vi "Get Heater.vi"(8 "error in (no error)":errorcluster, 9 "Heater Start Btn":refnum<vi>, 10 "Digital in":refnum<vi>, 11 "data":T1 {"Rotate_IND" items=["стоп", "Качалка Режим Авто", "Качалка Режим Ручной"]; "Termex_IND" items=["Термостат старт"=1, "Термостат стоп"=0]; "Mix_IND" items=["Мешалка движение вперёд"=1, "Мешалка движение назад"=2, "Мешалка стоп"=0]}) -> (0 "error out":errorcluster)   [LabVIEW 2023, in "GUI.lvlib" / "gui.lvclass"]
uses:
  gui.lvclass
  gui.lvclass/gui.ctl
  Modbus PLC/Modbus PLC/Data.ctl
  Modbus PLC/Modbus PLC/Modbus PLC.lvclass
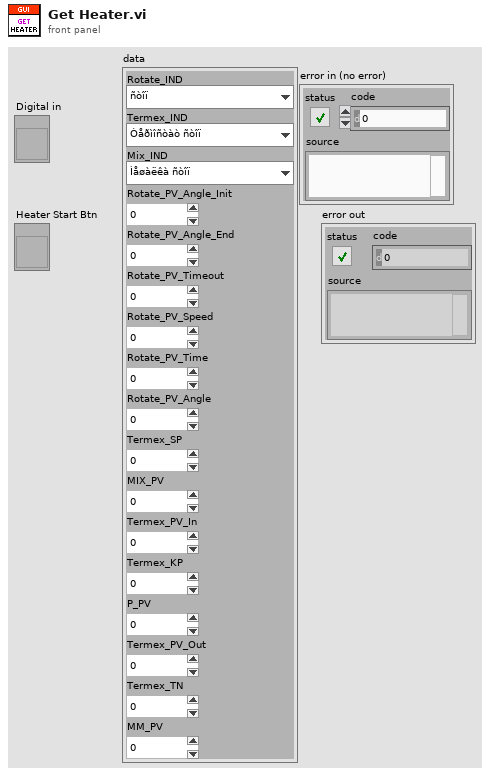
[diagram p1: front panel]
types:
  T1 = typedef "Modbus PLC.lvlib/Modbus PLC.lvclass/Data.ctl" = cluster{"Rotate_IND":u16, "Termex_IND":u16, "Mix_IND":u16, "Rotate_PV_Angle_Init":u16, "Rotate_PV_Angle_End":u16, "Rotate_PV_Timeout":u16, "Rotate_PV_Speed":u16, "Rotate_PV_Time":u16, "Rotate_PV_Angle":u16, "Termex_SP":sgl, "MIX_PV":u16, "Termex_PV_In":sgl, "Termex_KP":sgl, "P_PV":sgl, "Termex_PV_Out":sgl, "Termex_TN":sgl, "MM_PV":sgl}
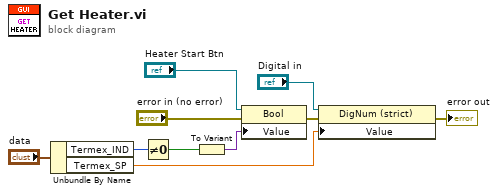
[diagram p0: block diagram]
diagram:
  n1 = Unbundle By Name("data") -> ("Termex_IND"=w9:u16, "Termex_SP"=w1:sgl)
  n2 = Not Equal To 0?(x=w9) -> (x != 0?=w7:bool)
  n3 = To Variant(anything=w7) -> (Variant=w6:variant)
  n4 = property class="Bool"(reference="Heater Start Btn", error in="error in (no error)", "Value"=w6) -> (error out=w4:errorcluster)  [unwired: 1 out]
  n5 = property class="DigNum (strict)"(reference="Digital in", error in=w4, "Value"=w1) -> (error out=→"error out":errorcluster)  [unwired: 1 out]
